vi "Fit Wavelength Data.vi"(10 "Numeric":i32, 11 "Array":dbl[](array[numeric])) -> (1 "Polynomial Coefficients":dbl[](array[numeric]), 2 "Best Polynomial Fit":dbl[](array[numeric]), 3 "XY Graph":cluster{"Ramp Pattern":dbl[], dbl[]}[](graph))   [LabVIEW 2020, in "Spectrometer Calibration.lvlib"]
uses:
  Spectrometer Calibration.lvlib
  <vilib>/Analysis/1siggen.llb/Ramp Pattern by Samples.vi
  <vilib>/Analysis/NI_AALPro.lvlib
  <vilib>/Analysis/NI_AALBase.lvlib
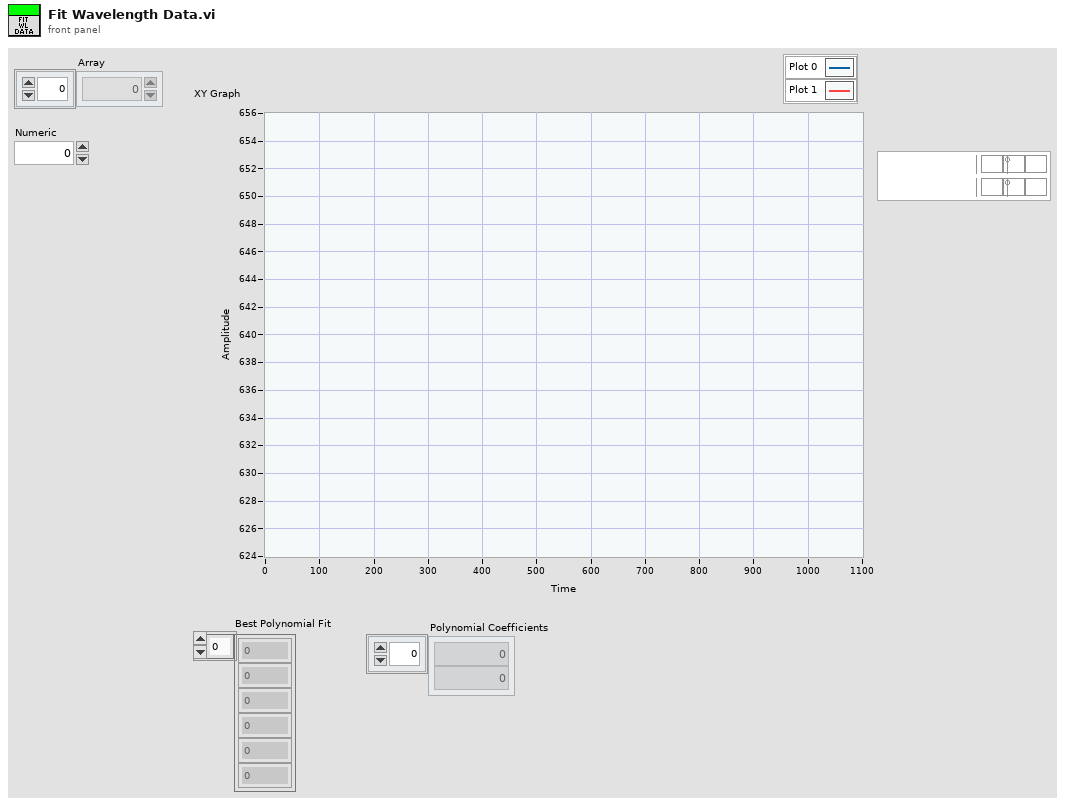
[diagram p1: front panel]
types:
  T1 = cluster{"Ramp Pattern":dbl[], "Best Polynomial Fit":dbl[]}
  T2 = cluster{"Ramp Pattern":dbl[], "Best Polynomial Fit":dbl[]}[]
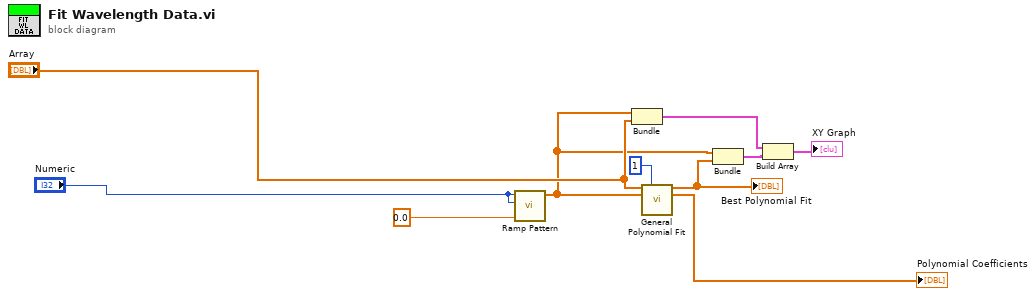
[diagram p0: block diagram]
diagram:
  n1 = call-poly <vilib>:"Ramp Pattern.vi"("start"=0.0, "end"="Numeric", "samples"="Numeric") -> ("Ramp Pattern"=w8:dbl[])  [unwired: 7 in, 1 out]
  n2 = Bundle("Ramp Pattern"=w8, "Array"="Array") -> (w9:cluster{"Ramp Pattern":dbl[], "Array":dbl[]})  [unwired: 1 in]
  n3 = call <vilib>:"General Polynomial Fit.vi"("Y"="Array", "polynomial order"=1, "X"=w8) -> ("Best Polynomial Fit"=w5:dbl[], "Polynomial Coefficients"=→"Polynomial Coefficients":dbl[])  [unwired: 9 in, 2 out]
  "Best Polynomial Fit" <- w5
  n4 = Bundle("Ramp Pattern"=w8, "Best Polynomial Fit"=w5) -> (w7:T1)  [unwired: 1 in]
  n5 = Build Array(w9, w7) -> (→"XY Graph":T2)
